vi "speed control.vi"(0 "flag":bool, 1 "Power":refnum<vi>, 2 "Speed":refnum<vi>, 3 "Pos":refnum<vi>, 4 "Dest":refnum<vi>, 5 "Enable 2":refnum<vi>, 6 "delay":dbl, 7 "Set Speed":dbl, 8 "Enable1":refnum<vi>, 9 "Deceletration":dbl, 10 "Accletration":dbl) -> ()   [LabVIEW 2017]
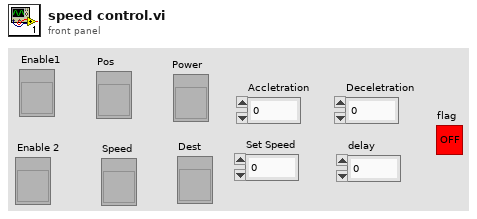
[diagram p1: front panel]
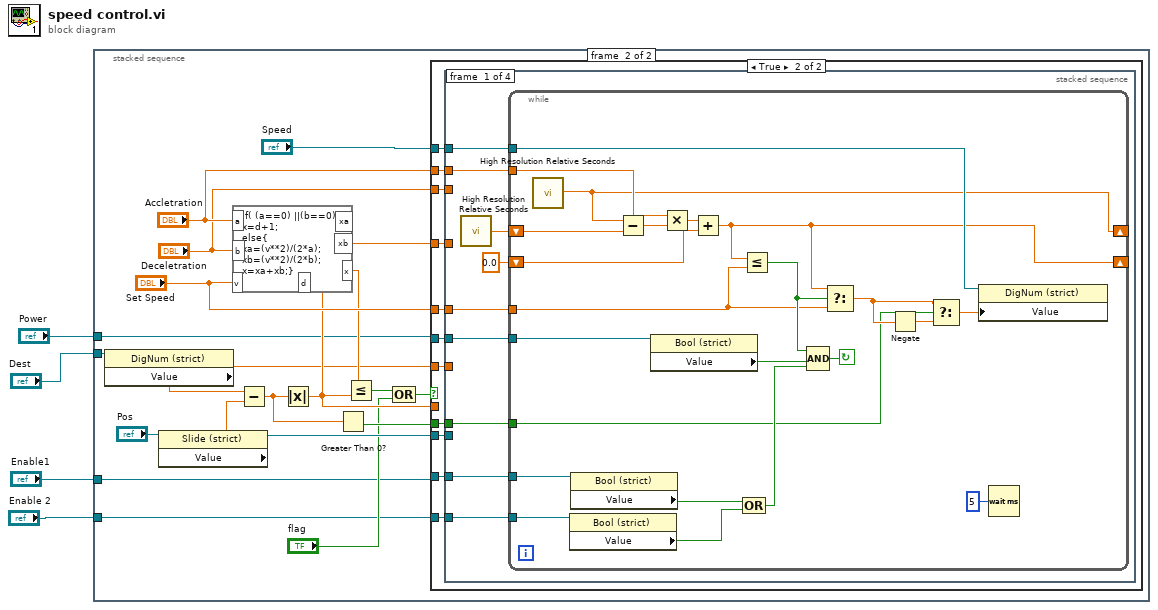
[diagram p0: block diagram]
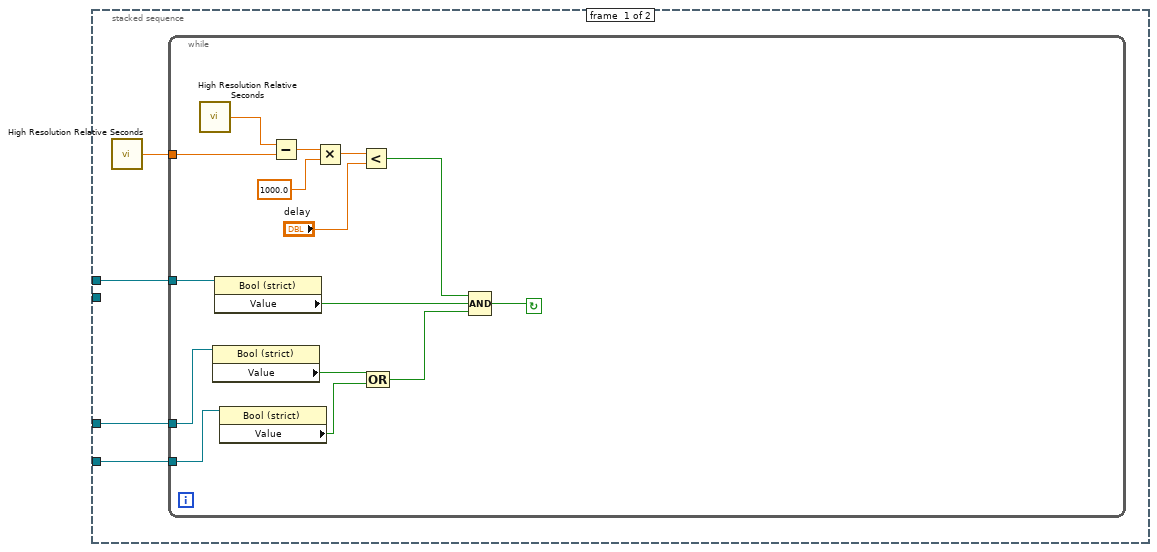
[diagram p2: hidden frame]
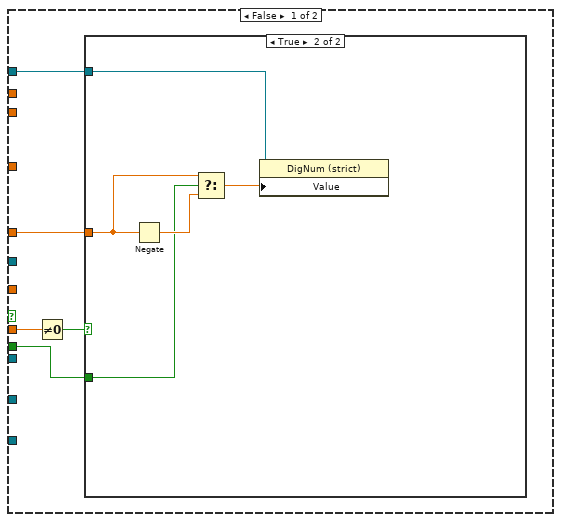
[diagram p3: hidden frame]
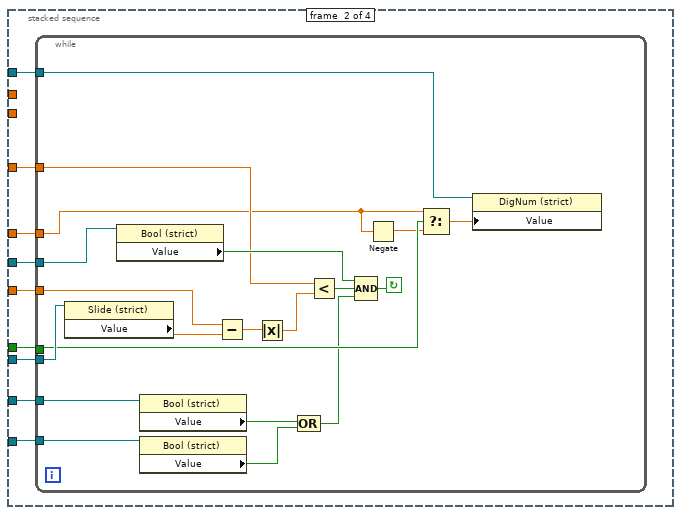
[diagram p5: hidden frame]
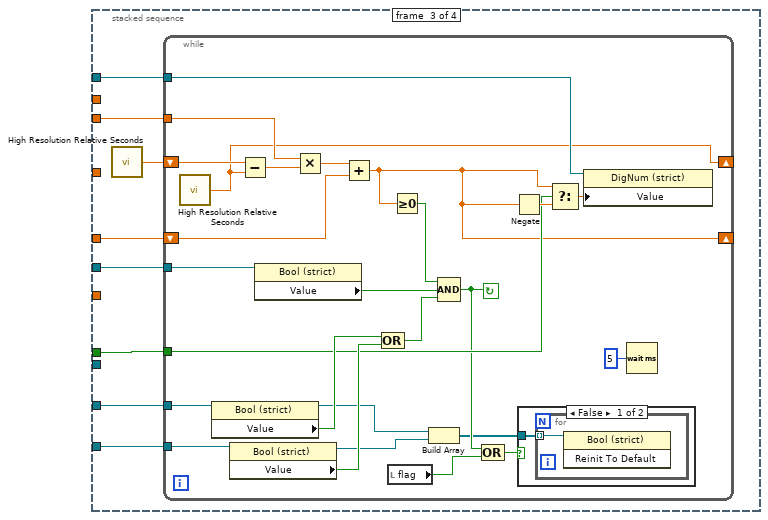
[diagram p6: hidden frame]
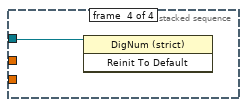
[diagram p8: hidden frame]
diagram:
  n1 = stacked-sequence {
    tunnel: "Enable1" -> [w6 w28]
    tunnel: "Enable 2" -> [w5 w27]
    tunnel: "Power" -> [w7 w26]
    tunnel: "Dest" -> [_ w25]
    frame #0 {
      n2 = call <vilib>:"High Resolution Relative Seconds.vi"() -> ("relative seconds"=w8:dbl)
      n3 = while {
        tunnel: w8 -> [w23]
        tunnel: w7 -> [w17]
        tunnel: w6 -> [w16]
        tunnel: w5 -> [w15]
        stop <- w9 continue-if-true
        n4 = call <vilib>:"High Resolution Relative Seconds.vi"() -> ("relative seconds"=w22:dbl)
        n5 = property class="Bool (strict)"(reference=w16) -> ("Value"=w14:bool)  [unwired: 1 in, 2 out]
        n6 = property class="Bool (strict)"(reference=w17) -> ("Value"=w12:bool)  [unwired: 1 in, 2 out]
        n7 = property class="Bool (strict)"(reference=w15) -> ("Value"=w13:bool)  [unwired: 1 in, 2 out]
        n8 = Subtract(x=w22, y=w23) -> (x-y=w21:dbl)
        n9 = Multiply(x=w21, y=1000.0) -> (x*y=w19:dbl)
        n10 = Less?(x=w19, y="delay") -> (x < y?=w10:bool)
        n11 = Compound Arithmetic op=OR(w14, w13) -> (w11:bool)
        n12 = Compound Arithmetic op=AND(w10, w12, w11) -> (w9:bool)
      }
    }
    frame #1 {
      n13 = property class="DigNum (strict)"(reference=w25) -> ("Value"=w24:dbl)  [unwired: 1 in, 2 out]
      n14 = property class="Slide (strict)"(reference="Pos") -> (reference out=w36:refnum<vi>, "Value"=w35:dbl)  [unwired: 1 in, 1 out]
      n15 = Subtract(x=w24, y=w35) -> (x-y=w34:dbl)
      n16 = Absolute Value(x=w34) -> (abs(x)=w33:dbl)
      n17 = formula code="if( (a==0) ||(b==0))\nx=d+1;\nelse{\nxa=(v**2)/(2*a);\nxb=(v**2)/(2*b);\nx=xa+xb;}"("a"="Accletration", "b"="Deceletration", "v"="Set Speed", "d"=w33) -> ("xb"=w41:dbl, "x"=w40:dbl)  [unwired: 1 out]
      n18 = Greater Than 0?(x=w34) -> (x > 0?=w30:bool)
      n19 = Less Or Equal?(x=w40, y=w33) -> (x <= y?=w32:bool)
      n20 = Compound Arithmetic op=OR(w32, "flag") -> (w31:bool)
      n21 = case shown="True" w31 {
        tunnel: "Speed" -> [w48 w61]
        tunnel: "Set Speed" -> [w47 w63]
        tunnel: "Accletration" -> [_ w64]
        tunnel: w26 -> [_ w62]
        tunnel: w36 -> [_ w60]
        tunnel: w24 -> [_ w59]
        tunnel: w41 -> [_ w58]
        tunnel: "Deceletration" -> [_ w57]
        tunnel: w28 -> [_ w56]
        tunnel: w27 -> [_ w55]
        tunnel: w33 -> [w45 _]
        tunnel: w30 -> [w44 w54]
        frame False {
          n22 = Not Equal To 0?(x=w45) -> (x != 0?=w46:bool)
          n23 = case shown="True" w46 {
            tunnel: w48 -> [_ w53]
            tunnel: w47 -> [_ w51]
            tunnel: w44 -> [_ w49]
            frame False {
            }
            frame True {
              n24 = Negate(x=w51) -> (-x=w50:dbl)
              n25 = Select(t=w51, s=w49, f=w50) -> (s? t:f=w52:dbl)
              n26 = property class="DigNum (strict)"(reference=w53, "Value"=w52) -> ()  [unwired: 1 in, 2 out]
            }
          }
        }
        frame True {
          n27 = stacked-sequence {
            tunnel: w64 -> [w72 _ _ _]
            tunnel: w63 -> [w71 w105 w127 _]
            tunnel: w62 -> [w70 w101 w131 _]
            tunnel: w61 -> [w69 w104 w132 w162]
            tunnel: w60 -> [_ w103 _ _]
            tunnel: w59 -> [_ w102 _ _]
            tunnel: w58 -> [_ w100 _ _]
            tunnel: w57 -> [_ _ w133 _]
            tunnel: w56 -> [w68 w99 w130 _]
            tunnel: w55 -> [w67 w98 w129 _]
            tunnel: w54 -> [w66 w97 w128 _]
            frame #0 {
              n28 = call <vilib>:"High Resolution Relative Seconds.vi"() -> ("relative seconds"=w73:dbl)
              n29 = while {
                tunnel: w72 -> [w93]
                tunnel: w71 -> [w90]
                tunnel: w70 -> [w92]
                tunnel: w69 -> [w91]
                tunnel: w68 -> [w86]
                tunnel: w67 -> [w85]
                tunnel: w66 -> [w80]
                shift-right: [w76] -> _
                shift-left: w73 -> [w79]
                shift-right: [w75] -> _
                shift-left: 0.0 -> [w77]
                stop <- w94 continue-if-true
                n30 = call <vilib>:"High Resolution Relative Seconds.vi"() -> ("relative seconds"=w76:dbl)
                n31 = property class="Bool (strict)"(reference=w85) -> ("Value"=w83:bool)  [unwired: 1 in, 2 out]
                n32 = property class="Bool (strict)"(reference=w86) -> ("Value"=w84:bool)  [unwired: 1 in, 2 out]
                n33 = Subtract(x=w76, y=w79) -> (x-y=w81:dbl)
                n34 = property class="Bool (strict)"(reference=w92) -> ("Value"=w95:bool)  [unwired: 1 in, 2 out]
                n35 = Multiply(x=w93, y=w81) -> (x*y=w78:dbl)
                n36 = Add(x=w78, y=w77) -> (x+y=w75:dbl)
                n37 = Less Or Equal?(x=w75, y=w90) -> (x <= y?=w96:bool)
                n38 = Compound Arithmetic op=OR(w84, w83) -> (w82:bool)
                n39 = Compound Arithmetic op=AND(w96, w95, w82) -> (w94:bool)
                n40 = Select(t=w75, s=w96, f=w90) -> (s? t:f=w87:dbl)
                n41 = Negate(x=w87) -> (-x=w88:dbl)
                n42 = Select(t=w87, s=w80, f=w88) -> (s? t:f=w89:dbl)
                n43 = property class="DigNum (strict)"(reference=w91, "Value"=w89) -> ()  [unwired: 1 in, 2 out]
                n44 = Wait (ms)(milliseconds to wait=u32 5) -> ()  [unwired: 1 out]
              }
            }
            frame #1 {
              n45 = while {
                tunnel: w105 -> [w111]
                tunnel: w104 -> [w125]
                tunnel: w103 -> [w124]
                tunnel: w102 -> [w123]
                tunnel: w101 -> [w121]
                tunnel: w100 -> [w117]
                tunnel: w97 -> [w113]
                tunnel: w99 -> [w110]
                tunnel: w98 -> [w109]
                stop <- w118 continue-if-true
                n46 = property class="Slide (strict)"(reference=w124) -> ("Value"=w122:dbl)  [unwired: 1 in, 2 out]
                n47 = property class="Bool (strict)"(reference=w121) -> ("Value"=w119:bool)  [unwired: 1 in, 2 out]
                n48 = property class="Bool (strict)"(reference=w110) -> ("Value"=w108:bool)  [unwired: 1 in, 2 out]
                n49 = property class="Bool (strict)"(reference=w109) -> ("Value"=w107:bool)  [unwired: 1 in, 2 out]
                n50 = Subtract(x=w123, y=w122) -> (x-y=w116:dbl)
                n51 = Absolute Value(x=w116) -> (abs(x)=w115:dbl)
                n52 = Compound Arithmetic op=OR(w108, w107) -> (w106:bool)
                n53 = Less?(x=w117, y=w115) -> (x < y?=w120:bool)
                n54 = Compound Arithmetic op=AND(w119, w120, w106) -> (w118:bool)
                n55 = Negate(x=w111) -> (-x=w112:dbl)
                n56 = Select(t=w111, s=w113, f=w112) -> (s? t:f=w114:dbl)
                n57 = property class="DigNum (strict)"(reference=w125, "Value"=w114) -> ()  [unwired: 1 in, 2 out]
              }
            }
            frame #2 {
              n58 = call <vilib>:"High Resolution Relative Seconds.vi"() -> ("relative seconds"=w126:dbl)
              n59 = while {
                tunnel: w133 -> [w159]
                tunnel: w132 -> [w157]
                tunnel: w131 -> [w156]
                tunnel: w130 -> [w151]
                tunnel: w129 -> [w150]
                tunnel: w128 -> [w146]
                shift-right: [w137] -> _
                shift-left: w126 -> [w145]
                shift-right: [w135] -> _
                shift-left: w127 -> [w136]
                stop <- w142 continue-if-true
                n60 = call <vilib>:"High Resolution Relative Seconds.vi"() -> ("relative seconds"=w137:dbl)
                n61 = property class="Bool (strict)"(reference=w151) -> (reference out=w144:refnum<vi>, "Value"=w149:bool)  [unwired: 1 in, 1 out]
                n62 = property class="Bool (strict)"(reference=w150) -> (reference out=w143:refnum<vi>, "Value"=w148:bool)  [unwired: 1 in, 1 out]
                n63 = Subtract(x=w145, y=w137) -> (x-y=w138:dbl)
                n64 = property class="Bool (strict)"(reference=w156) -> ("Value"=w155:bool)  [unwired: 1 in, 2 out]
                n65 = Multiply(x=w159, y=w138) -> (x*y=w158:dbl)
                n66 = Add(x=w158, y=w136) -> (x+y=w135:dbl)
                n67 = Compound Arithmetic op=OR(w149, w148) -> (w147:bool)
                n68 = local read "flag"() -> (w141:bool)
                n69 = Greater Or Equal To 0?(x=w135) -> (x >= 0?=w154:bool)
                n70 = Build Array(w144, w143) -> (w140:refnum<vi>[])
                n71 = Compound Arithmetic op=AND(w154, w155, w147) -> (w142:bool)
                n72 = Compound Arithmetic op=OR(w142, w141) -> (w139:bool)
                n73 = Negate(x=w135) -> (-x=w152:dbl)
                n74 = case shown="False" w139 {
                  tunnel: w140 -> [w160 _]
                  frame False {
                    n75 = for {
                      tunnel: w160 -> [w161] mode=indexing
                      n76 = invoke class="Bool (strict)" method="Reinit To Default"(reference=w161) -> ()  [unwired: 2 in, 3 out]
                    }
                  }
                  frame True {
                  }
                }
                n77 = Select(t=w135, s=w146, f=w152) -> (s? t:f=w153:dbl)
                n78 = property class="DigNum (strict)"(reference=w157, "Value"=w153) -> ()  [unwired: 1 in, 2 out]
                n79 = Wait (ms)(milliseconds to wait=u32 5) -> ()  [unwired: 1 out]
              }
            }
            frame #3 {
              n80 = invoke class="DigNum (strict)" method="Reinit To Default"(reference=w162) -> ()  [unwired: 2 in, 3 out]
            }
          }
        }
      }
    }
  }
